vi "Open View FP.vi"(0 "GUI Container Actor in":refnum<class "GUI Container Actor.lvclass">, 1 "Activate on Open (F)":bool, 5 "View":string, 7 "View Hierarchy Level":i32, 11 "error in (no error)":errorcluster, 12 "State On Open (Standard)":T1(ring)=enum."Standard") -> (4 "GUI Container Actor out":refnum<class "GUI Container Actor.lvclass">, 15 "error out":errorcluster)   [LabVIEW 2017, in "GUI Views.lvlib" / "GUI Container Actor.lvclass"]
doc: "Opens the Front Panel of a specified Actor Core VI of the the specified View class hierarchy. The Front Panel is specified by: \n\n<b> View </b> String theat contains the name of the View\n\n<b> View Hierarchy Level</b> the level on the subclassing hierarchy of the GUI View actor, it is used to choose the Actor Core Front Panel among all the exisiting sublcasses of the GUI VIew Actor present in the View specified above"
uses:
  GUI Container Actor.lvclass
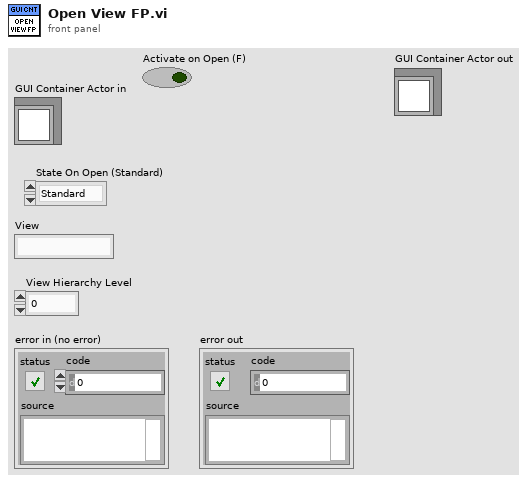
[diagram p1: front panel]
types:
  T1 = enum32{"Invalid", "Standard", "Closed", "Hidden", "Minimized", "Maximized"}
  T2 = typedef "GUI Views.lvlib/GUI Container Actor.lvclass/View Status.ctl" = cluster{"View Details":T3, "Front Panel Statuses":T4[]}
  T3 = typedef "GUI Views.lvlib/GUI Container Actor.lvclass/View Details.ctl" = cluster{"Enqueuer":refnum<class "Message Enqueuer.lvclass">, "VI References":refnum<vi>[], "FP References":refnum<vi>[]}
  T4 = typedef "GUI Views.lvlib/GUI Container Actor.lvclass/FP Status.ctl" = cluster{"FP Open":bool, "Inserted in Subpanel":bool, "Subpanel":string}
  T5 = typedef "GUI Views.lvlib/GUI Container Actor.lvclass/VI References.ctl" = cluster{"FP Ref":refnum<vi>, "VI Ref":refnum<vi>}
  T6 = typedef "GUI Views.lvlib/GUI Container Actor.lvclass/Subpanel Status.ctl" = cluster{"Subpanel Ref":refnum<vi>, "Inserted View":string, "Inserted View Hierarchy Level":i32}
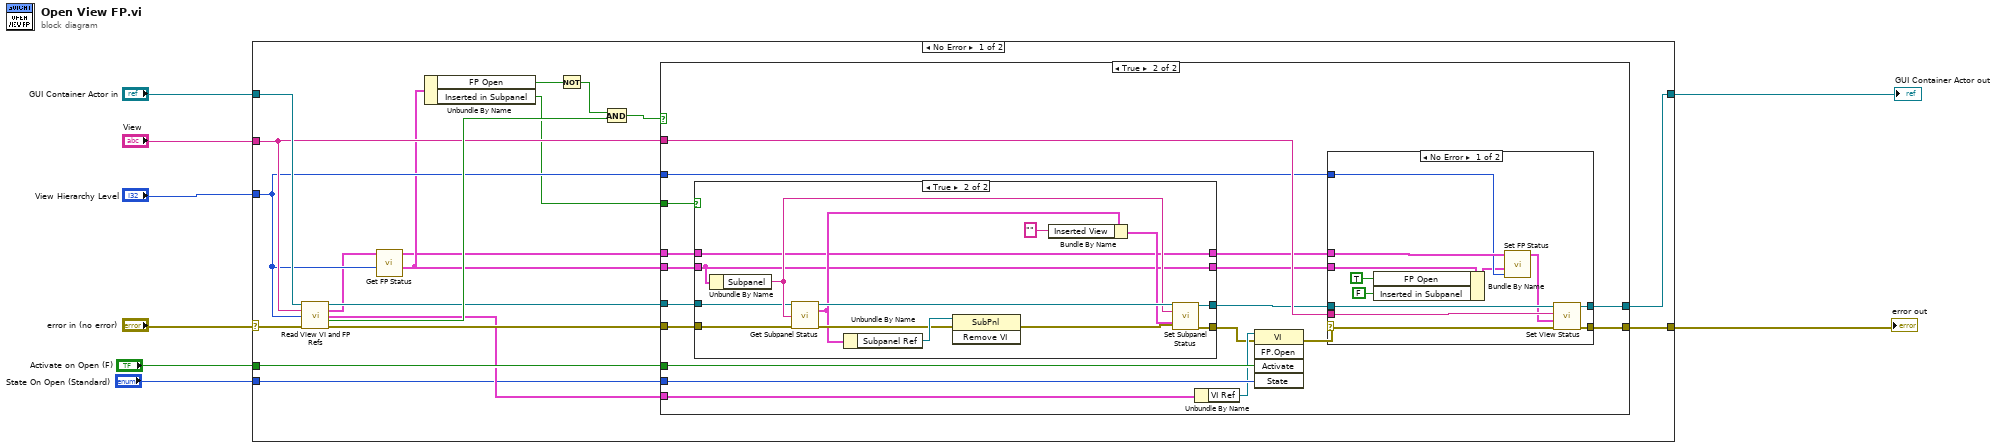
[diagram p0: block diagram]
diagram:
  n1 = case shown="No Error" "error in (no error)" {
    selector: "error in (no error)" -> [w26 w80]
    tunnel: [w27 w80] -> w8
    tunnel: "GUI Container Actor in" -> [w24 w81]
    tunnel: "View Hierarchy Level" -> [w14 _]
    tunnel: "View" -> [w17 _]
    tunnel: [w16 w81] -> w3
    tunnel: "State On Open (Standard)" -> [w15 _]
    tunnel: "Activate on Open (F)" -> [w20 _]
    frame No Error {
      n2 = call "Read View VI and FP Refs.vi"("GUI Container Actor in"=w24, "View"=w17, "View Hierarchy Level"=w14, "error in (no error)"=w26) -> ("GUI Container Actor out"=w18:refnum<class "GUI Container Actor.lvclass">, "View Status"=w12:T2, "VI References"=w19:T5, "View Found"=w22:bool, "error out"=w25:errorcluster)  [unwired: 7 in]
      n3 = call "Get FP Status.vi"("View Hierarchy Level"=w14, "View Status in"=w12) -> ("FP Status"=w13:T4, "View Status out"=w11:T2)  [unwired: 8 in]
      n4 = Unbundle By Name(w13) -> ("FP Open"=w23:bool, "Inserted in Subpanel"=w9:bool)
      n5 = Not(x=w23) -> (.not. x?=w10:bool)
      n6 = Compound Arithmetic op=AND(w10, w22) -> (w21:bool)
      n7 = case shown="True" w21 {
        tunnel: [w29 w42] -> w27
        tunnel: w15 -> [_ w46]
        tunnel: w25 -> [w29 w37]
        tunnel: w20 -> [_ w47]
        tunnel: w19 -> [_ w45]
        tunnel: w18 -> [w28 w34]
        tunnel: w17 -> [_ w41]
        tunnel: [w28 w40] -> w16
        tunnel: w13 -> [_ w35]
        tunnel: w11 -> [_ w31]
        tunnel: w14 -> [_ w39]
        tunnel: w9 -> [_ w38]
        frame False {
        }
        frame True {
          n8 = case shown="True" w38 {
            tunnel: w37 -> [w50 w57]
            tunnel: [w50 w56] -> w36
            tunnel: w35 -> [w48 w53]
            tunnel: w34 -> [w51 w55]
            tunnel: [w51 w54] -> w33
            tunnel: [w48 w53] -> w32
            tunnel: w31 -> [w49 w52]
            tunnel: [w49 w52] -> w30
            frame False {
            }
            frame True {
              n9 = Unbundle By Name(w53) -> ("Subpanel"=w61:string)
              n10 = call "Get Subpanel Status.vi"("GUI Container Actor in"=w55, "Subpanel"=w61, "error in (no error)"=w57) -> ("GUI Container Actor out"=w62:refnum<class "GUI Container Actor.lvclass">, "Subpanel Status"=w60:T6, "error out"=w64:errorcluster)  [unwired: 9 in, 1 out]
              n11 = Unbundle By Name(w60) -> ("Subpanel Ref"=w65:refnum<vi>)
              n12 = invoke class="SubPnl" method="Remove VI"(reference=w65, error in=w64) -> (error out=w58:errorcluster)  [unwired: 1 in, 2 out]
              n13 = Bundle By Name(cluster=w60, "Inserted View"="") -> (w59:T6)
              n14 = call "Set Subpanel Status.vi"("GUI Container Actor in"=w62, "Subpanel"=w61, "Subpanel Status"=w59, "error in (no error)"=w58) -> ("GUI Container Actor out"=w54:refnum<class "GUI Container Actor.lvclass">, "error out"=w56:errorcluster)  [unwired: 9 in, 1 out]
            }
          }
          n15 = Unbundle By Name(w45) -> ("VI Ref"=w44:refnum<vi>)
          n16 = invoke class="VI" method="FP.Open"(reference=w44, error in=w36, "Activate"=w47, "State"=w46) -> (error out=w43:errorcluster)  [unwired: 1 in, 4 out]
          n17 = case shown="No Error" w43 {
            selector: w43 -> [w75 w79]
            tunnel: [w77 w79] -> w42
            tunnel: w33 -> [w76 w78]
            tunnel: w41 -> [w73 _]
            tunnel: [w72 w78] -> w40
            tunnel: w32 -> [w71 _]
            tunnel: w30 -> [w70 _]
            tunnel: w39 -> [w69 _]
            frame No Error {
              n18 = Bundle By Name(cluster=w71, "FP Open"=TRUE, "Inserted in Subpanel"=FALSE) -> (w67:T4)
              n19 = call "Set FP Status.vi"("View Hierarchy Level"=w69, "FP Status"=w67, "View Status in"=w70) -> ("View Status out"=w68:T2)  [unwired: 8 in]
              n20 = call "Set View Status.vi"("error in (no error)"=w75, "View Status"=w68, "View"=w73, "GUI Container Actor in"=w76) -> ("error out"=w77:errorcluster, "GUI Container Actor out"=w72:refnum<class "GUI Container Actor.lvclass">)  [unwired: 5 in, 1 out]
            }
            frame Error {
            }
          }
        }
      }
    }
    frame Error {
    }
  }
  "error out" <- w8
  "GUI Container Actor out" <- w3
